vi "AOL Properties bundler-DBL.vi"(7 "Keys setup.DBL":T2, 8 "error in (no error)":errorcluster, 9 "Section name":string="AOL Properties", 10 "AOL Properties":T3={"AOD 1 thickness (mm)"=0.0, "AOD 2 thickness (mm)"=0.0, "AOD 3 thickness (mm)"=0.0, "AOD 4 thickness (mm)"=0.0, "AOD 5 thickness (mm)"=0.0, "AOD 6 thickness (mm)"=0.0, "AOD 1-2 separation (mm)"=0.0, "AOD 2-3 separation (mm)"=0.0, "AOD 3-4 separation (mm)"=0.0, "AOD 4-5 separation (mm)"=0.0, "AOD 5-6 separation (mm)"=0.0, "AOD 1 X Offset"=0.0, "AOD 2 X Offset"=0.0, "AOD 3 X Offset"=0.0, "AOD 4 X Offset"=0.0, "AOD 1 Y Offset"=0.0, "AOD 2 Y Offset"=0.0, "AOD 3 Y Offset"=0.0, "AOD 4 Y Offset"=1.0, "AOD 1 X Direction"=0.0, "AOD 2 X Direction"=0.0, "AOD 3 X Direction"=0.0, "AOD 4 X Direction"=0.0, "AOD 1 Y Direction"=1.0, "AOD 2 Y Direction"=0.0, "AOD 3 Y Direction"=0.0023, "AOD 4 Y Direction"=0.0046, "AOD 1 Centre (mm)"=0.0, "AOD 2 Centre (mm)"=0.0, "AOD 3 Centre (mm)"=0.0, "AOD 4 Centre (mm)"=0.0, "Timing Offset AOD 1"=0.0, "Timing Offset AOD 2"=0.0, "Timing Offset AOD 3"=0.0, "Timing Offset AOD 4"=0.0, "AOD Optical offset 1"=20000.0, "AOD Optical offset 2"=20000.0, "AOL aperture (mm)"=15.0, "AOL centre wavelength (nm)"=1.0, "AOL centre frequency (MHz)"=1.0, "Diffraction mode"=1.0, "Crystal length (mm)"=0.0, "Acoustic velocity (m/s)"=1.0, "Pair deflection ratio"=1.0, "AOD fill time (us)"=1.0, "AOD Ord. Refractive index"=2.22, "AOD ExtraOrd. Refractive index"=2.22}, 11 "Refnum in":T1) -> (0 "error out":errorcluster, 2 "AOL Properties":T3={"AOD 1 thickness (mm)"=0.0, "AOD 2 thickness (mm)"=0.0, "AOD 3 thickness (mm)"=0.0, "AOD 4 thickness (mm)"=0.0, "AOD 5 thickness (mm)"=0.0, "AOD 6 thickness (mm)"=0.0, "AOD 1-2 separation (mm)"=0.0, "AOD 2-3 separation (mm)"=0.0, "AOD 3-4 separation (mm)"=0.0, "AOD 4-5 separation (mm)"=0.0, "AOD 5-6 separation (mm)"=0.0, "AOD 1 X Offset"=0.0, "AOD 2 X Offset"=0.0, "AOD 3 X Offset"=0.0, "AOD 4 X Offset"=0.0, "AOD 1 Y Offset"=0.0, "AOD 2 Y Offset"=0.0, "AOD 3 Y Offset"=0.0, "AOD 4 Y Offset"=1.0, "AOD 1 X Direction"=0.0, "AOD 2 X Direction"=0.0, "AOD 3 X Direction"=0.0, "AOD 4 X Direction"=0.0, "AOD 1 Y Direction"=1.0, "AOD 2 Y Direction"=0.0, "AOD 3 Y Direction"=0.0023, "AOD 4 Y Direction"=0.0046, "AOD 1 Centre (mm)"=0.0, "AOD 2 Centre (mm)"=0.0, "AOD 3 Centre (mm)"=0.0, "AOD 4 Centre (mm)"=0.0, "Timing Offset AOD 1"=0.0, "Timing Offset AOD 2"=0.0, "Timing Offset AOD 3"=0.0, "Timing Offset AOD 4"=0.0, "AOD Optical offset 1"=20000.0, "AOD Optical offset 2"=20000.0, "AOL aperture (mm)"=15.0, "AOL centre wavelength (nm)"=1.0, "AOL centre frequency (MHz)"=1.0, "Diffraction mode"=1.0, "Crystal length (mm)"=0.0, "Acoustic velocity (m/s)"=1.0, "Pair deflection ratio"=1.0, "AOD fill time (us)"=1.0, "AOD Ord. Refractive index"=2.22, "AOD ExtraOrd. Refractive index"=2.22}, 3 "Refnum out":T1)   [LabVIEW 2017]
uses:
  Typedefs/AOL Properties Cluster.ctl
  Typedefs/Ini file interface (DBL).ctl
  <vilib>/Utility/config.llb/Config Data RefNum.ctl
  <vilib>/Utility/config.llb/NI_LVConfig.lvlib
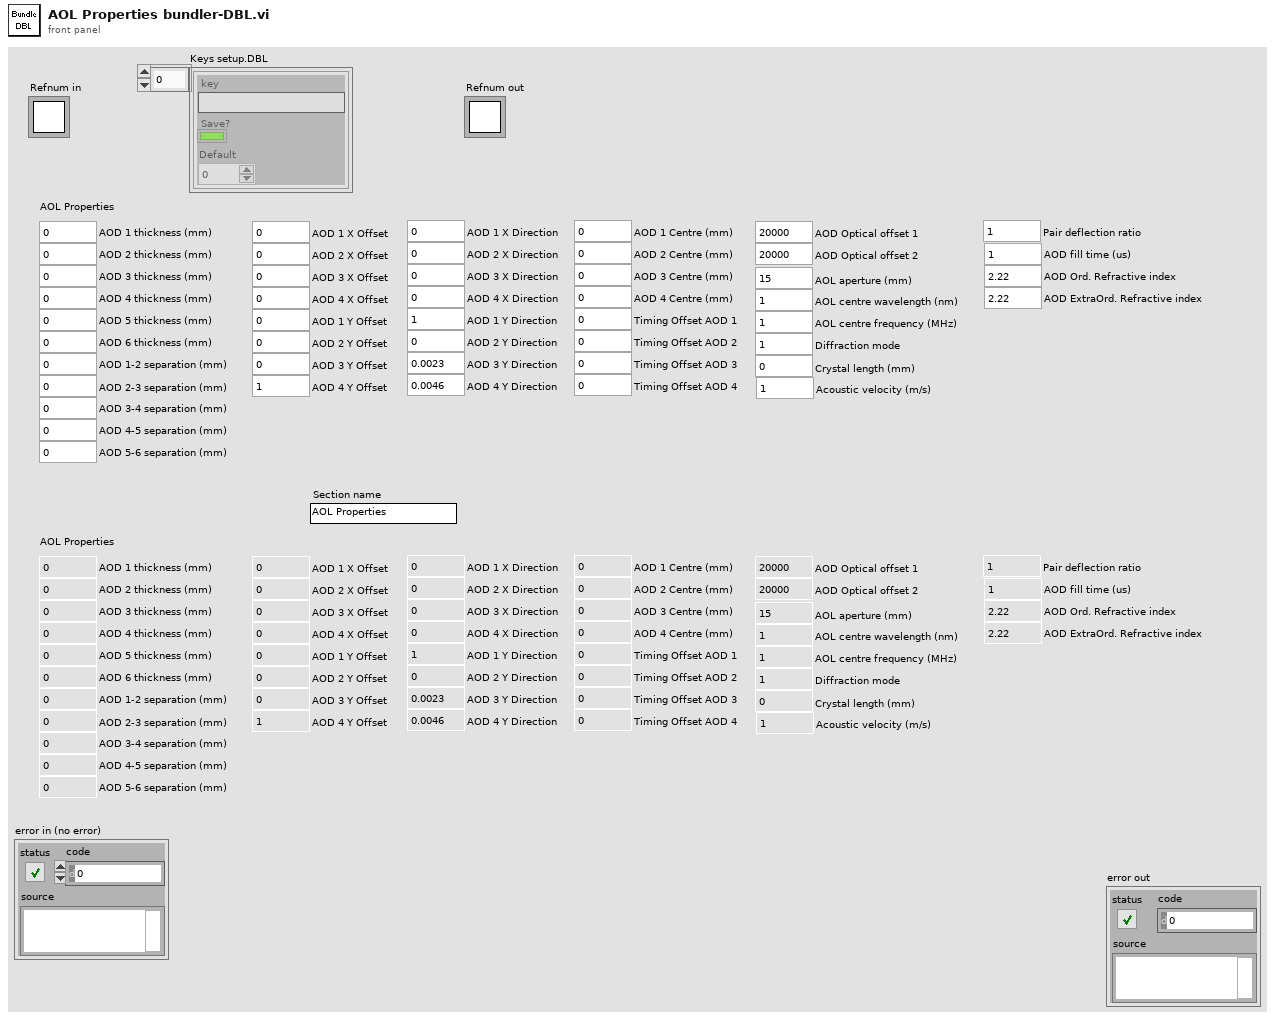
[diagram p1: front panel]
types:
  T1 = typedef "NI_LVConfig.lvlib/Config Data RefNum.ctl" = refnum<k1>
  T2 = typedef "Ini file interface (DBL).ctl" = cluster{"key":string, "Save?":bool, "Default":dbl}[]
  T3 = typedef "AOL Properties Cluster.ctl" = cluster{"AOD 1 thickness (mm)":dbl, "AOD 2 thickness (mm)":dbl, "AOD 3 thickness (mm)":dbl, "AOD 4 thickness (mm)":dbl, "AOD 5 thickness (mm)":dbl, "AOD 6 thickness (mm)":dbl, "AOD 1-2 separation (mm)":dbl, "AOD 2-3 separation (mm)":dbl, "AOD 3-4 separation (mm)":dbl, "AOD 4-5 separation (mm)":dbl, "AOD 5-6 separation (mm)":dbl, "AOD 1 X Offset":dbl, "AOD 2 X Offset":dbl, "AOD 3 X Offset":dbl, "AOD 4 X Offset":dbl, "AOD 1 Y Offset":dbl, "AOD 2 Y Offset":dbl, "AOD 3 Y Offset":dbl, "AOD 4 Y Offset":dbl, "AOD 1 X Direction":dbl, "AOD 2 X Direction":dbl, "AOD 3 X Direction":dbl, "AOD 4 X Direction":dbl, "AOD 1 Y Direction":dbl, "AOD 2 Y Direction":dbl, "AOD 3 Y Direction":dbl, "AOD 4 Y Direction":dbl, "AOD 1 Centre (mm)":dbl, "AOD 2 Centre (mm)":dbl, "AOD 3 Centre (mm)":dbl, "AOD 4 Centre (mm)":dbl, "Timing Offset AOD 1":dbl, "Timing Offset AOD 2":dbl, "Timing Offset AOD 3":dbl, "Timing Offset AOD 4":dbl, "AOD Optical offset 1":dbl, "AOD Optical offset 2":dbl, "AOL aperture (mm)":dbl, "AOL centre wavelength (nm)":dbl, "AOL centre frequency (MHz)":dbl, "Diffraction mode":dbl, "Crystal length (mm)":dbl, "Acoustic velocity (m/s)":dbl, "Pair deflection ratio":dbl, "AOD fill time (us)":dbl, "AOD Ord. Refractive index":dbl, "AOD ExtraOrd. Refractive index":dbl}
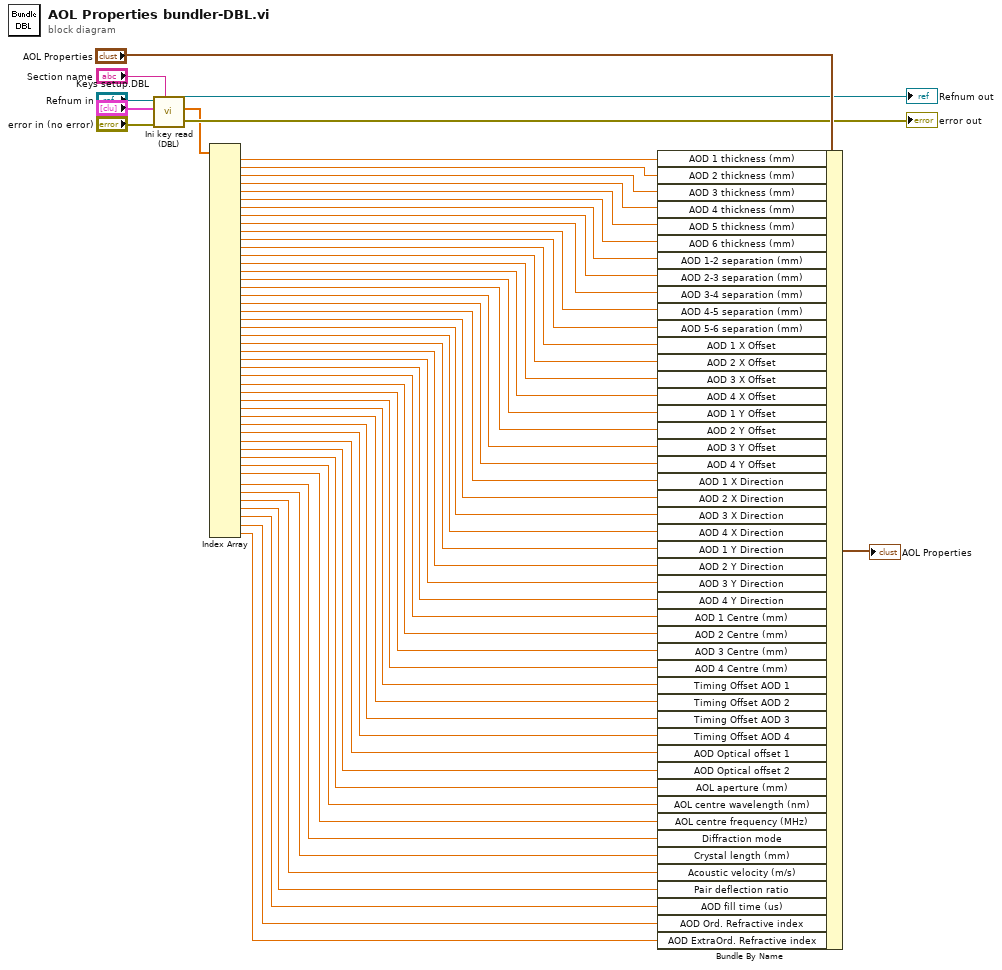
[diagram p0: block diagram]
diagram:
  n1 = call "Ini key read (DBL).vi"("Section name"="Section name", "error in (no error)"="error in (no error)", "Parameter names & setup"="Keys setup.DBL", "Ini file refnum in"="Refnum in") -> ("error out"=→"error out":errorcluster, "Value read/used"=w49:dbl[], "Ini file refnum out"=→"Refnum out":T1)  [unwired: 5 in]
  n2 = Index Array(array=w49) -> (element #1=w48:dbl, element #2=w47:dbl, element #3=w46:dbl, element #4=w45:dbl, element #5=w44:dbl, element #6=w43:dbl, element #7=w42:dbl, element #8=w41:dbl, element #9=w40:dbl, element #10=w39:dbl, element #11=w38:dbl, element #12=w37:dbl, element #13=w36:dbl, element #14=w35:dbl, element #15=w34:dbl, element #16=w33:dbl, element #17=w32:dbl, element #18=w31:dbl, element #19=w30:dbl, element #20=w29:dbl, element #21=w28:dbl, element #22=w27:dbl, element #23=w26:dbl, element #24=w25:dbl, element #25=w24:dbl, element #26=w23:dbl, element #27=w22:dbl, element #28=w21:dbl, element #29=w20:dbl, element #30=w19:dbl, element #31=w18:dbl, element #32=w17:dbl, element #33=w16:dbl, element #34=w15:dbl, element #35=w14:dbl, element #36=w13:dbl, element #37=w12:dbl, element #38=w11:dbl, element #39=w10:dbl, element #40=w9:dbl, element #41=w8:dbl, element #42=w7:dbl, element #43=w6:dbl, element #44=w5:dbl, element #45=w4:dbl, element #46=w3:dbl, element #47=w2:dbl)  [unwired: 47 in]
  n3 = Bundle By Name(cluster="AOL Properties", "AOD 1 thickness (mm)"=w48, "AOD 2 thickness (mm)"=w47, "AOD 3 thickness (mm)"=w46, "AOD 4 thickness (mm)"=w45, "AOD 5 thickness (mm)"=w44, "AOD 6 thickness (mm)"=w43, "AOD 1-2 separation (mm)"=w42, "AOD 2-3 separation (mm)"=w41, "AOD 3-4 separation (mm)"=w40, "AOD 4-5 separation (mm)"=w39, "AOD 5-6 separation (mm)"=w38, "AOD 1 X Offset"=w37, "AOD 2 X Offset"=w36, "AOD 3 X Offset"=w35, "AOD 4 X Offset"=w34, "AOD 1 Y Offset"=w33, "AOD 2 Y Offset"=w32, "AOD 3 Y Offset"=w31, "AOD 4 Y Offset"=w30, "AOD 1 X Direction"=w29, "AOD 2 X Direction"=w28, "AOD 3 X Direction"=w27, "AOD 4 X Direction"=w26, "AOD 1 Y Direction"=w25, "AOD 2 Y Direction"=w24, "AOD 3 Y Direction"=w23, "AOD 4 Y Direction"=w22, "AOD 1 Centre (mm)"=w21, "AOD 2 Centre (mm)"=w20, "AOD 3 Centre (mm)"=w19, "AOD 4 Centre (mm)"=w18, "Timing Offset AOD 1"=w17, "Timing Offset AOD 2"=w16, "Timing Offset AOD 3"=w15, "Timing Offset AOD 4"=w14, "AOD Optical offset 1"=w13, "AOD Optical offset 2"=w12, "AOL aperture (mm)"=w11, "AOL centre wavelength (nm)"=w10, "AOL centre frequency (MHz)"=w9, "Diffraction mode"=w8, "Crystal length (mm)"=w7, "Acoustic velocity (m/s)"=w6, "Pair deflection ratio"=w5, "AOD fill time (us)"=w4, "AOD Ord. Refractive index"=w3, "AOD ExtraOrd. Refractive index"=w2) -> (→"AOL Properties":T3)
